vi "Write.vi"(8 "error in (no error)":errorcluster, 10 "Boolean 1D":T1[](array[typedef]), 11 "Boolean in":refnum<class "Abs_Boolean_1D.lvclass">) -> (0 "error out":errorcluster, 3 "Boolean out":refnum<class "Abs_Boolean_1D.lvclass">)   [LabVIEW 2021, in "Abs_Boolean_1D.lvclass"]
uses:
  Abs_Boolean_1D.lvclass
  Support/Element Type.ctl
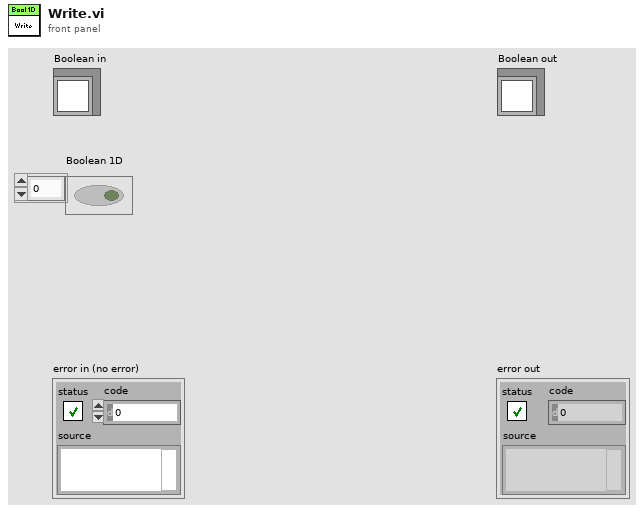
[diagram p1: front panel]
types:
  T1 = typedef "Abs_Boolean_1D.lvclass/Element Type.ctl" = bool
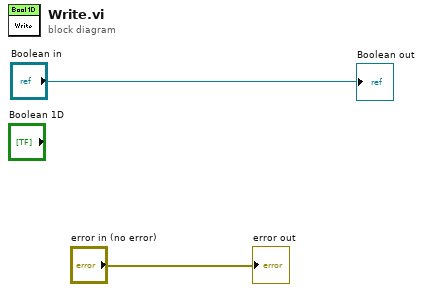
[diagram p0: block diagram]
diagram:
  "error out" <- "error in (no error)"
  "Boolean out" <- "Boolean in"
